vi "AddNodeAutoName.vi"(8 "error in (no error)":errorcluster, 9 "Default Node Name":string, 10 "point":cluster{"x":i16, "y":i16}, 11 "FSM in":refnum<class "FSM.Graph.lvclass">) -> (0 "error out":errorcluster, 2 "Name":string, 3 "FSM out":refnum<class "FSM.Graph.lvclass">)   [LabVIEW 2015, in "FSM.Graph.lvclass"]
uses:
  FSM.Graph.lvclass
  FSM.Graph.lvclass/FSM.Graph.ctl
  FSM.Node/FSM.Node.lvclass/FSM.Node.ctl
  FSM.Node/Shape.ctl
  FSM.Node/Read Name.vi
  FSM.Node/Write Shape.vi
  FSM.Node/FSM.Node.lvclass
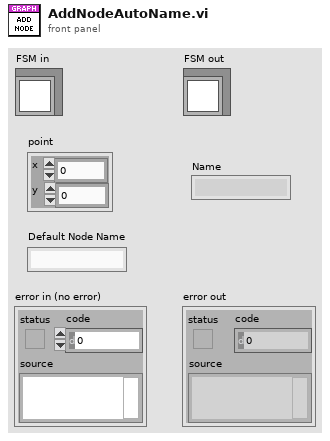
[diagram p1: front panel]
types:
  T1 = typedef "FSM.Node.lvclass/Shape.ctl" = enum16{"Default", "Start", "Action", "End"}
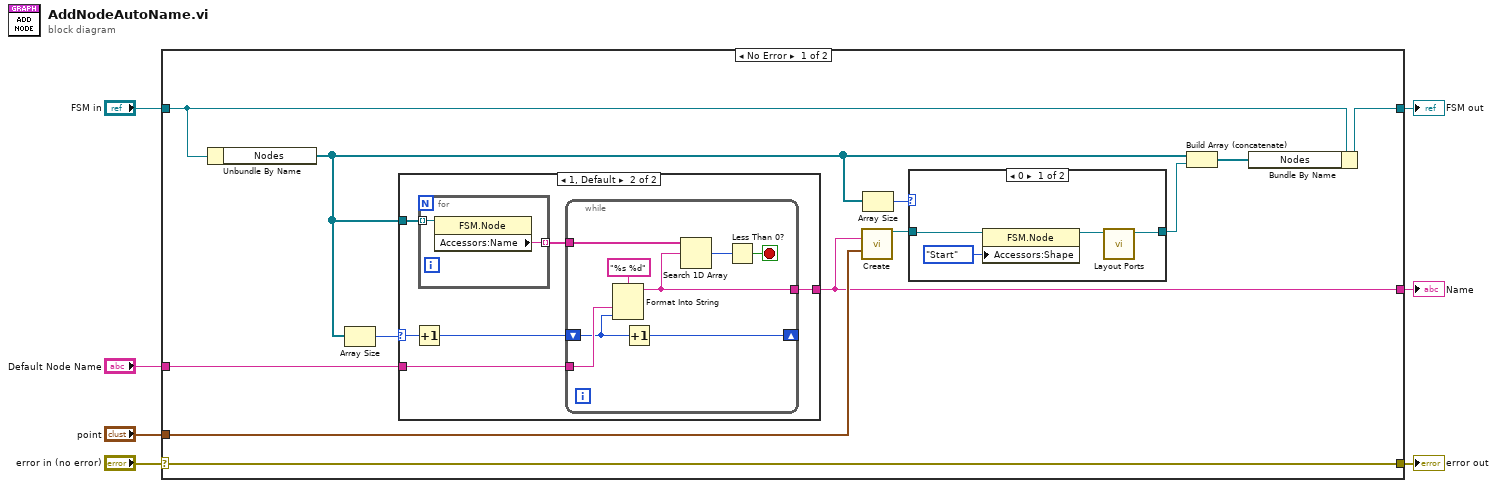
[diagram p0: block diagram]
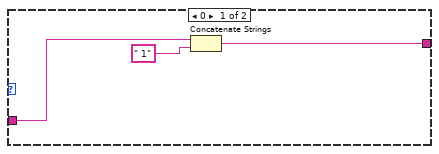
[diagram p3: hidden frame]
diagram:
  n1 = case shown="No Error" "error in (no error)" {
    selector: "error in (no error)" -> [w19 w45]
    tunnel: [w19 w45] -> w6
    tunnel: [w16 w44] -> w4
    tunnel: "FSM in" -> [w18 w44]
    tunnel: "Default Node Name" -> [w14 _]
    tunnel: "point" -> [w17 _]
    tunnel: [w12 _] -> w1
    frame No Error {
      n2 = Unbundle By Name(w18) -> ("Nodes"=w11:refnum<class "FSM.Node.lvclass">[])
      n3 = Array Size(array=w11) -> (size(s)=w13:i32)
      n4 = case shown="1, Default" w13 {
        selector: w13 -> [_ w32]
        tunnel: w11 -> [_ w33]
        tunnel: w14 -> [w27 w29]
        tunnel: [w26 w28] -> w12
        frame 0 {
          n5 = Concatenate Strings(w27, " 1" ("string")) -> (w26:string)
        }
        frame 1, Default {
          n6 = Increment(x=w32) -> (x+1=w31:i32)
          n7 = for {
            tunnel: w33 -> [w43] mode=indexing
            tunnel: [w42] -> w30 mode=indexing
            n8 = property class="FSM.Node"(reference=w43) -> ("Accessors:Name"=w42:string)  [unwired: 1 in, 2 out]
          }
          n9 = while {
            shift-right: [w39] -> _
            shift-left: w31 -> [w38]
            tunnel: w30 -> [w37]
            tunnel: w29 -> [w40]
            tunnel: [w34] -> w28
            stop <- w35 stop-if-true
            n10 = Format Into String(format string="%s %d", w40, w38) -> (resulting string=w34:string)  [unwired: 2 in, 1 out]
            n11 = Increment(x=w38) -> (x+1=w39:i32)
            n12 = Search 1D Array(1D array=w37, element=w34) -> (index of element=w36:i32)  [unwired: 1 in]
            n13 = Less Than 0?(x=w36) -> (x < 0?=w35:bool)
          }
        }
      }
      n14 = call "Create.vi"("Name"=w12, "Center"=w17) -> ("FSM.Node"=w10:refnum<class "FSM.Node.lvclass">)  [unwired: 13 in]
      n15 = Array Size(array=w11) -> (size(s)=w9:i32)
      n16 = case shown="0" w9 {
        tunnel: w10 -> [w23 w24]
        tunnel: [w20 w24] -> w8
        frame 0 {
          n17 = property class="FSM.Node"(reference=w23, "Accessors:Shape"=Shape."Start" ("Shape")) -> (reference out=w21:refnum<class "FSM.Node.lvclass">)  [unwired: 1 in, 1 out]
          n18 = call "Layout Ports.vi"("Node in"=w21) -> ("Node out"=w20:refnum<class "FSM.Node.lvclass">)  [unwired: 9 in, 1 out]
        }
        frame 1, Default {
        }
      }
      n19 = Build Array (concatenate)(w11, w8) -> (w15:refnum<class "FSM.Node.lvclass">[])
      n20 = Bundle By Name(cluster=w18, "Nodes"=w15) -> (w16:refnum<class "FSM.Graph.lvclass">)
    }
    frame Error {
    }
  }
  "error out" <- w6
  "FSM out" <- w4
  "Name" <- w1
